vi "Add Panel Layout.vi"(4 "subpanel UIDs":i32[](array[numeric]), 6 "subpanel refnums":refnum<vi>[](array[refnum]), 8 "error in":errorcluster, 9 "panel layout":refnum<class "VI Panel Layout.lvclass">, 10 "VI ref":refnum<vi>, 11 "state in":T1) -> (0 "error out":errorcluster, 1 "VI info index":i32, 3 "state out":T1)   [LabVIEW 2010, in "NI_SE_Config Front Panel Layout.lvlib"]
uses:
  NI_SE_Config Front Panel Layout.lvlib
  State.ctl
  VI Info.ctl
  VI Panel Layout/VI Panel Layout.lvclass
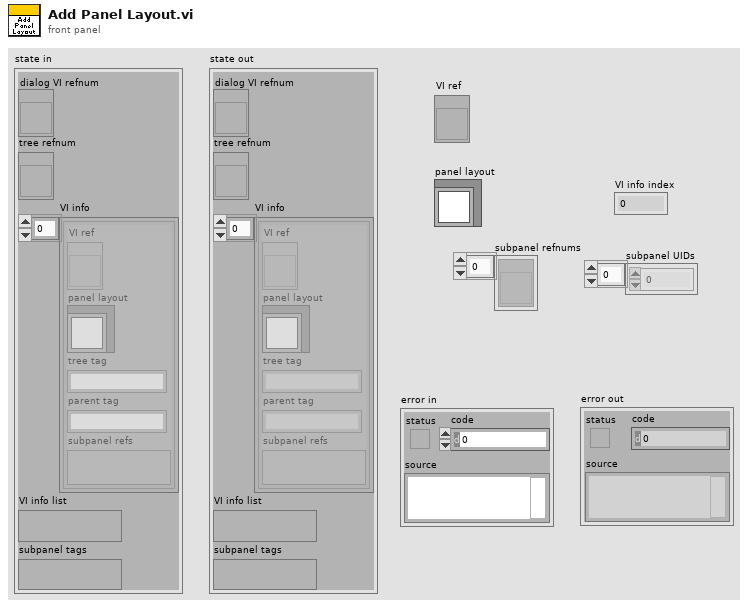
[diagram p1: front panel]
types:
  T1 = typedef "NI_SE_Config Front Panel Layout.lvlib/State.ctl" = cluster{"dialog VI refnum":refnum<vi>, "tree refnum":refnum<vi>, "VI info":T2[], "VI info list":variant, "subpanel tags":variant}
  T2 = typedef "NI_SE_Config Front Panel Layout.lvlib/VI Info.ctl" = cluster{"VI ref":refnum<vi>, "panel layout":refnum<class "VI Panel Layout.lvclass">, "tree tag":string, "parent tag":string, "subpanel refs":variant}
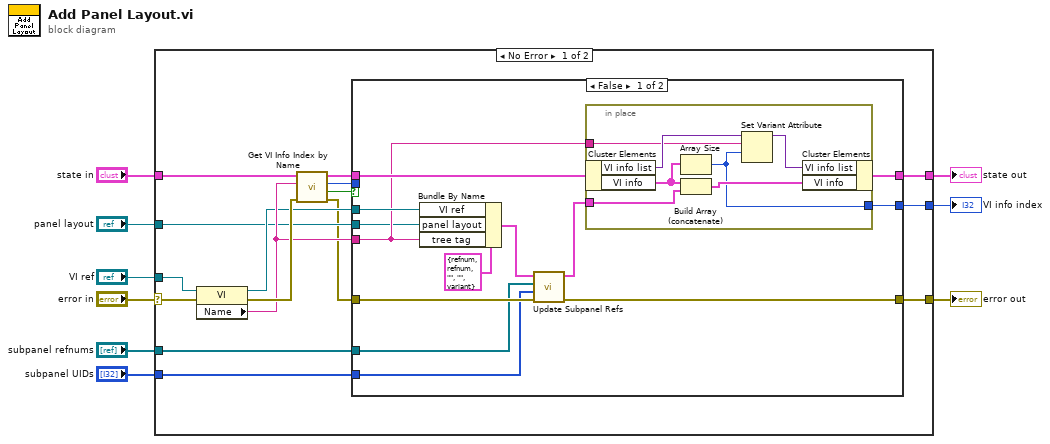
[diagram p0: block diagram]
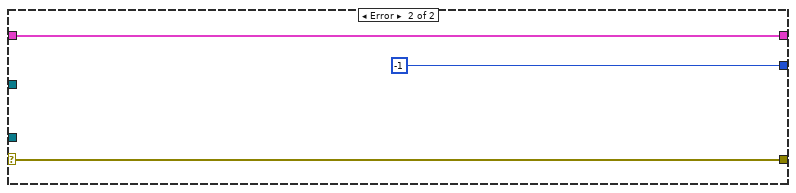
[diagram p3: hidden frame]
diagram:
  n1 = case shown="No Error" "error in" {
    selector: "error in" -> [w19 w50]
    tunnel: "state in" -> [w20 w51]
    tunnel: [w16 w51] -> w7
    tunnel: [w14 w50] -> w6
    tunnel: "VI ref" -> [w18 _]
    tunnel: "panel layout" -> [w17 _]
    tunnel: "subpanel refnums" -> [w13 _]
    tunnel: "subpanel UIDs" -> [w12 _]
    tunnel: [w10 -1 ("VI info index")] -> w1
    frame No Error {
      n2 = property class="VI"(reference=w18, error in=w19) -> (reference out=w21:refnum<vi>, error out=w24:errorcluster, "Name"=w23:string)
      n3 = call "Get VI Info Index by Name.vi"("error in"=w24, "VI name"=w23, "state in"=w20) -> ("error out"=w15:errorcluster, "found?"=w25:bool, "VI info index"=w11:i32, "state out"=w22:T1)  [unwired: 5 in]
      n4 = case shown="False" w25 {
        tunnel: w21 -> [w37 _]
        tunnel: [w36 w48] -> w16
        tunnel: w22 -> [w35 w48]
        tunnel: w23 -> [w34 _]
        tunnel: w17 -> [w33 _]
        tunnel: w15 -> [w32 w47]
        tunnel: [w31 w47] -> w14
        tunnel: w13 -> [w28 _]
        tunnel: w12 -> [w27 _]
        tunnel: w11 -> [_ w46]
        tunnel: [w26 w46] -> w10
        frame False {
          n5 = Bundle By Name(cluster=T2 {"VI ref"=refnum, "panel layout"=refnum, "tree tag"="", "parent tag"="", "subpanel refs"=variant} ("VI tree information"), "VI ref"=w37, "panel layout"=w33, "tree tag"=w34) -> (w30:T2)
          n6 = call "Update Subpanel Refs.vi"("error in"=w32, "subpanel UIDs"=w27, "subpanel refnums"=w28, "VI info in"=w30) -> ("error out"=w31:errorcluster, "VI info out"=w29:T2)  [unwired: 6 in]
          n7 = in-place {
            in-place-border: w29 -> [w44]
            in-place-border: w34 -> [w40]
            in-place-border: [w39] -> w26
            n8 = in-place-cluster #1(w35) -> ("VI info list"=w42:variant, "VI info"=w43:T2[])
            n9 = Array Size(array=w43) -> (size(s)=w39:i32)
            n10 = Build Array (concatenate)(w43, w44) -> (w45:T2[])
            n11 = Set Variant Attribute(Variant=w42, name=w40, value=w39) -> (Variant out=w41:variant)  [unwired: 1 in, 2 out]
            n12 = in-place-cluster #1("VI info list"=w41, "VI info"=w45) -> (w36:T1)
          }
        }
        frame True {
          # "VI has already been added."
        }
      }
    }
    frame Error {
    }
  }
  "state out" <- w7
  "error out" <- w6
  "VI info index" <- w1
